vi "TrajectorySystem.vi"() -> ()   [LabVIEW 2025]
panel:
  out "TrajectorySystem/done":bool caption="Done"
  out "TrajectorySystem/ElapsedTrajTime":dbl caption="Elapsed Time" format="%12.1f"
  out "TrajectorySystem/rotErr":dbl caption="Rotational Error" format="%11.2f"
  out "TrajectorySystem/yErr":dbl caption="Y Error" format="%11.2f"
  out "TrajectorySystem/timeLengthOfTrajectory":dbl caption="Total Time" format="%12.1f"
  out "TrajectorySystem/xErr":dbl caption="X Error" format="%11.2f"
  out "TrajectorySystem/onTarget":bool caption="On Target"
  # "TRAJECTORY"
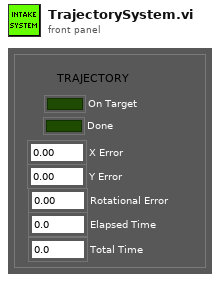
[diagram p1: front panel]
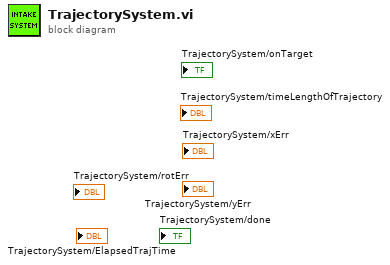
[diagram p0: block diagram]
diagram:
